vi "VMP_subvi_teststand.vi"() -> ()   [LabVIEW 2016]
uses:
  <vilib>/vision/driver/NI_Vision_Acquisition_Software.lvlib
panel:
  out "Current stage position [mm]":cluster{"X":dbl, "Y":dbl, "Z":dbl}
  out "moving":bool
  out "error out":errorcluster
  in  "Calibrated positions of fiducials [mm]":dbl[][](array[numeric])
  in  "Camera Name":refnum<k21>="cam0" caption="IMAQdx Session"
  out "Current field of view":T1(plugin-control)
  out "Module Progress Report":T2(array[cluster])
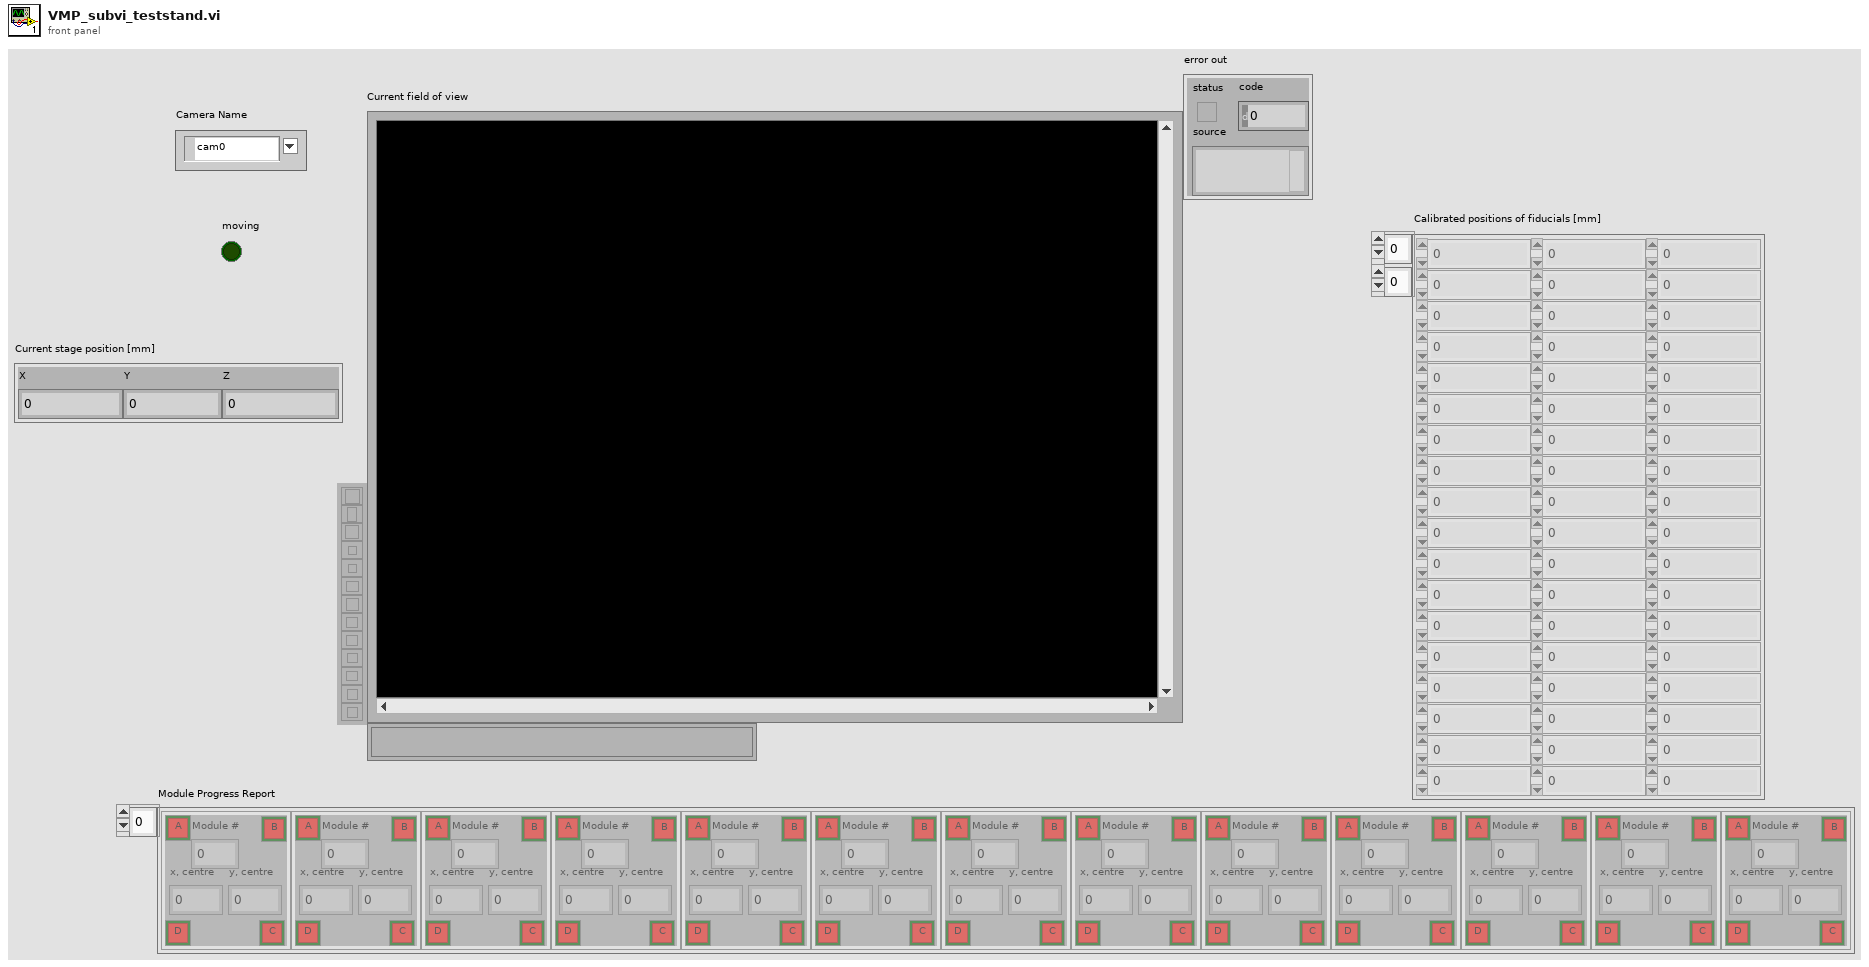
[diagram p1: front panel]
types:
  T1 = typedef "IMAQ Image.ctl" = refnum<image>
  T2 = cluster{"A":bool, "x, centre":dbl, "y, centre":dbl, "Module #":i32, "B":bool, "D":bool, "C":bool}[]
  T3 = enum16{"Mark C", "Mark B", "Strip Corner", "[None]"}
  T4 = typedef "IMAQdx.ctl" = refnum<k21>
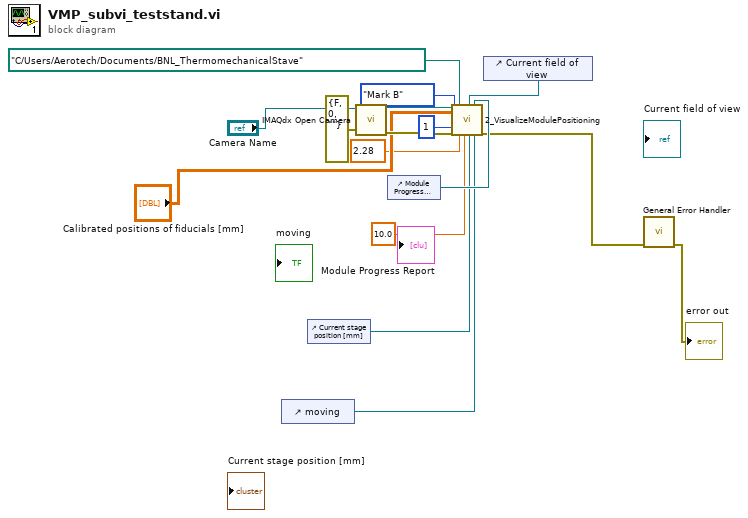
[diagram p0: block diagram]
diagram:
  n1 = control-ref of="moving"() -> (w1:refnum<vi>)
  n2 = control-ref of="Current stage position [mm]"() -> (w2:refnum<vi>)
  n3 = call <vilib>:"IMAQdx Open Camera.vi"("error in"=errorcluster {"status"=FALSE, "code"=0, "source"=""}, "Session In"="Camera Name") -> ("error out"=w11:errorcluster, "Session Out"=w16:T4)  [unwired: 1 in, 7 out]
  n4 = control-ref of="Module Progress Report"() -> (w13:refnum<vi>)
  n5 = control-ref of="Current field of view"() -> (w12:refnum<vi>)
  n6 = call "2_VisualizeModulePositioning.vi"("Session in"=w16, "Calibrated positions of fiducials [mm]"="Calibrated positions of fiducials [mm]", "Module fiducial marker"=T3."Mark B", "N modules"=1, "error in (no error)"=w11, "Templates path"=path "C:/Users/Aerotech/Documents/BNL_ThermomechanicalStave", "Calibration [um/pix]"=2.28, "Placement tolerance [um]"=10.0, "Current Image"=w12, "Current stage position"=w2, "Module Report"=w13, "Moving"=w1) -> ("error out"=w9:errorcluster)  [unwired: 6 in, 1 out]
  n7 = call <vilib>:"General Error Handler.vi"("error in (no error)"=w9) -> ("error out"=→"error out":errorcluster)  [unwired: 10 in, 4 out]
